vi "Add Multiple.vi"(7 "Settings":T2, 8 "error in (no error)":errorcluster, 9 "Fixtures":T1[](array[typedef]), 10 "Routine":T3[](array[typedef]), 11 "Assembly in":refnum<class "Assembly Run.lvclass">) -> (0 "error out":errorcluster, 3 "Assembly out":refnum<class "Assembly Run.lvclass">)   [LabVIEW 2021, in "Assembly Run.lvclass"]
uses:
  Assembly Run.lvclass
  Routine/Routine Enum.ctl
  Routine/Settings.ctl
  Workspace/Fixture Enum.ctl
  Routine/Routine.lvclass
  Workspace/Fixture.lvclass
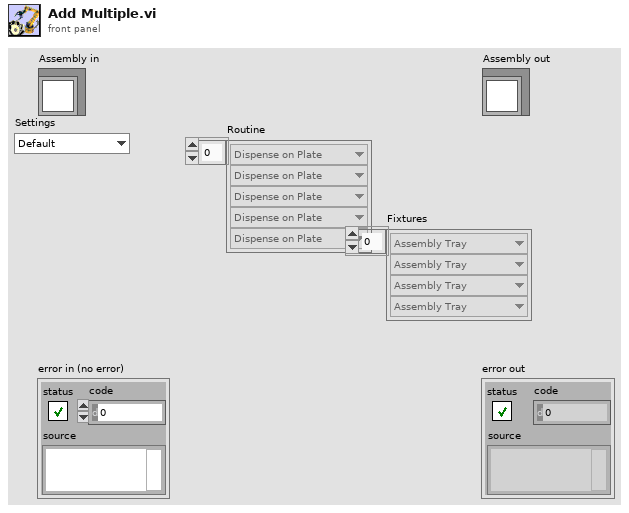
[diagram p1: front panel]
types:
  T1 = typedef "Fixture.lvclass/Fixture Enum.ctl" = enum16{"Assembly Tray", "Syringe Space", "Component", "Pick Up Tool", "Current Position"}
  T2 = typedef "Routine.lvclass/Settings.ctl" = enum16{"Default", "Custom"}
  T3 = typedef "Routine.lvclass/Routine Enum.ctl" = enum16{"Primary Pick Up", "Secondary Pick Up", "Put Down All", "Secure Syringe", "Release Syringe", "Dispense on Plate", "Dispense on Sensor", "Pick Up All", "Put Down Secondary", "Dispense on Kapton"}
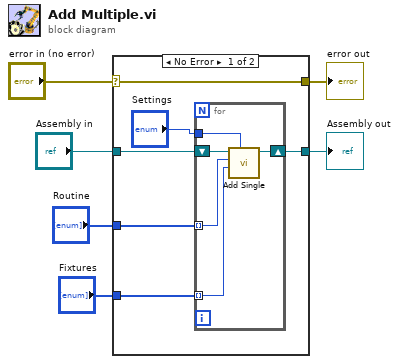
[diagram p0: block diagram]
diagram:
  n1 = case shown="No Error" "error in (no error)" {
    selector: "error in (no error)" -> [w12 w19]
    tunnel: [w12 w19] -> w5
    tunnel: [w10 w18] -> w3
    tunnel: "Assembly in" -> [w11 w18]
    tunnel: "Routine" -> [w9 _]
    tunnel: "Fixtures" -> [w7 _]
    frame No Error {
      n2 = for {
        shift-right: [w14] -> w10
        shift-left: w11 -> [w16]
        tunnel: w9 -> [w13] mode=indexing
        tunnel: "Settings" -> [w15]
        tunnel: w7 -> [w17] mode=indexing
        n3 = call-dynamic "Add Single.vi"("Settings"=w15, "Fixture"=w17, "Routine"=w13, "UI in"=w16) -> ("UI out"=w14:refnum<class "Assembly Run.lvclass">)  [unwired: 5 in, 1 out]
      }
    }
    frame Error {
    }
  }
  "error out" <- w5
  "Assembly out" <- w3
